vi "Initialize.vi"(8 "error in (no error)":errorcluster, 11 "BL-Retract-Cmd in":refnum<class "BL-Retract-Cmd.lvclass">) -> (0 "error out":errorcluster, 3 "BL-Retract-Cmd out":refnum<class "BL-Retract-Cmd.lvclass">)   [LabVIEW 2013, in "BL-Retract-Cmd.lvclass"]
uses:
  BL-Retract-Cmd.lvclass
  States/BL-Retracting-State/BL-Retracting-State.lvclass
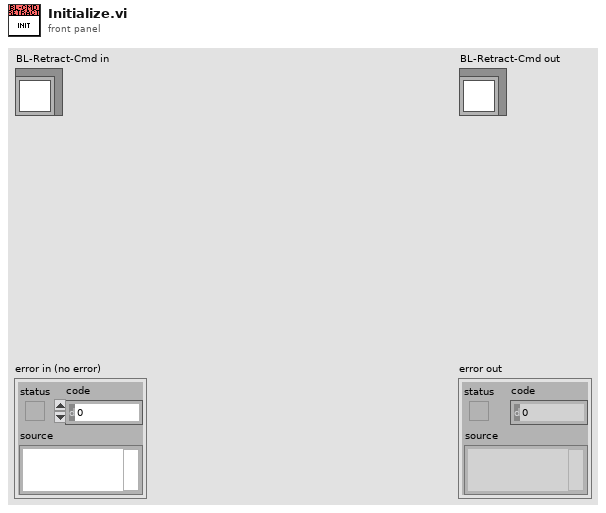
[diagram p1: front panel]
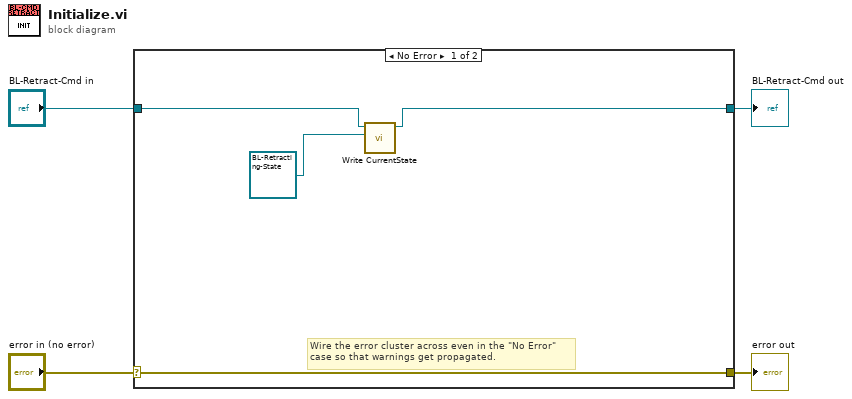
[diagram p0: block diagram]
diagram:
  n1 = case shown="No Error" "error in (no error)" {
    selector: "error in (no error)" -> [w8 w10]
    tunnel: [w8 w10] -> w3
    tunnel: [w6 w9] -> w1
    tunnel: "BL-Retract-Cmd in" -> [w7 w9]
    frame No Error {
      # "Wire the error cluster across even in the \"No Error\"\ncase so that warnings get propagated."
      n2 = call-dynamic "Write CurrentState.vi"("State.lvclass"=refnum<class "BL-Retracting-State.lvclass"> refnum ("BL-Retracting-State.lvclass"), "Command in"=w7) -> ("Command out"=w6:refnum<class "BL-Retract-Cmd.lvclass">)  [unwired: 8 in, 1 out]
    }
    frame Error {
    }
  }
  "error out" <- w3
  "BL-Retract-Cmd out" <- w1
